vi "Emballage_BDD_Display PDF in Dialog LV2009.vi"(0 "PDF file":path, 5 "error in (no error)":errorcluster) -> (19 "error out":errorcluster)   [LabVIEW 2020]
doc: "Use this VI to display a PDF document in a dialog box.\nIn the <B>PDF file</B> text box, enter the path to the PDF you want to display, or click the <B>Browse</B> button to navigate to a file.\nClick the <B>Run</B> button to view the PDF in the <B>PDF display</B>.\nClick the <B>Stop</B> button to stop the VI and remove the PDF from display."
panel:
  in  "Imprimer":bool caption="Blank"
  in  "Stop":bool
  out "chaîne résultante":string
  in  "AcroPDF":refnum<k7>(container)
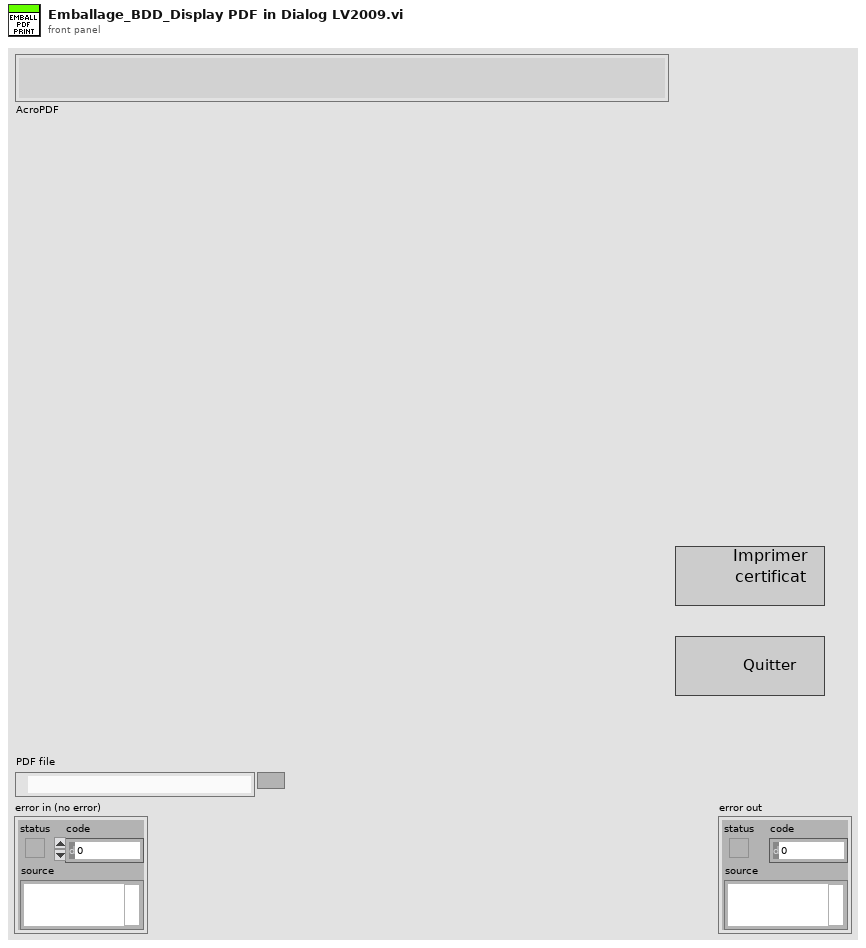
[diagram p1: front panel]
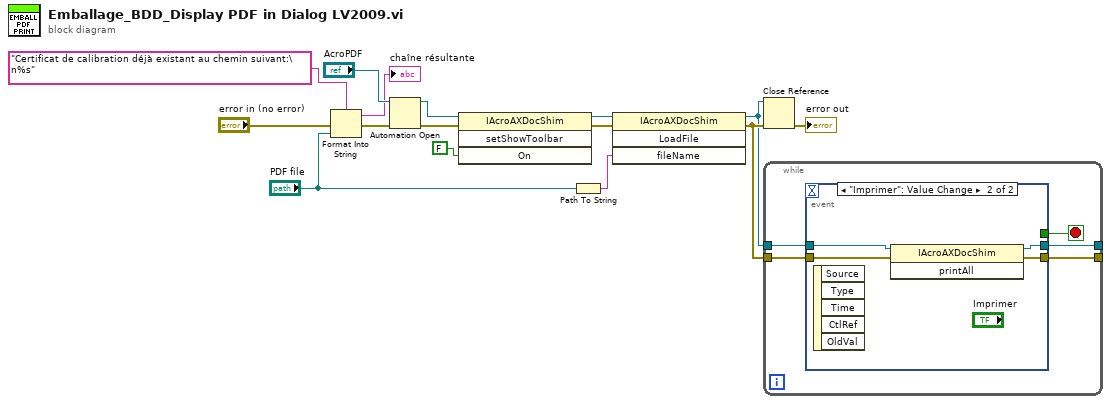
[diagram p0: block diagram]
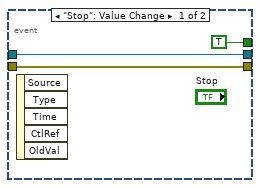
[diagram p2: hidden frame]
diagram:
  n1 = Format Into String(format string="Certificat de calibration déjà existant au chemin suivant:\n%s" ("Message"), error in="error in (no error)", "PDF file") -> (resulting string=→"chaîne résultante":string, error out=w4:errorcluster)  [unwired: 1 in]
  n2 = Automation Open(error in (no error)=w4, Automation Refnum="AcroPDF") -> (Automation Refnum=w10:refnum<k7>, error out=w9:errorcluster)  [unwired: 2 in]
  n3 = invoke class="IAcroAXDocShim" method="setShowToolbar"(reference=w10, error in=w9, "On"=FALSE) -> (reference out=w13:refnum<k7>, error out=w12:errorcluster)  [unwired: 1 in, 2 out]
  n4 = Path To String(path="PDF file") -> (string=w15:string)
  n5 = invoke class="IAcroAXDocShim" method="LoadFile"(reference=w13, error in=w12, "fileName"=w15) -> (reference out=w1:refnum<k7>, error out=w2:errorcluster)  [unwired: 1 in, 2 out]
  n6 = Close Reference(reference=w1, error in (no error)=w2) -> (error out=→"error out":errorcluster)
  n7 = while {
    tunnel: w1 -> [w19]
    tunnel: [w18] -> _
    tunnel: [w17] -> _
    tunnel: w2 -> [w16]
    stop <- w20 stop-if-true
    n8 = event shown="[1] \"Imprimer\": Value Change" {
      selector: _ -> [_ _]
      dyn-events: _ -> [_ _]
      timeout: _ -> [_ _]
      tunnel: [TRUE _] -> w20
      tunnel: w19 -> [w21 w27]
      tunnel: [w21 w26] -> w18
      tunnel: [w22 w25] -> w17
      tunnel: w16 -> [w22 w24]
      event "Stop": Value Change {
        n9 = event-data() -> ()  [unwired: 1 in, 5 out]
      }
      event "Imprimer": Value Change {
        n10 = event-data() -> ()  [unwired: 1 in, 5 out]
        n11 = invoke class="IAcroAXDocShim" method="printAll"(reference=w27, error in=w24) -> (reference out=w26:refnum<k7>, error out=w25:errorcluster)  [unwired: 1 in, 1 out]
      }
    }
  }
